vi "LineStyle_GetObjectStatus.vi"(0 "reference":refnum<class "LineStyle.lvclass">, 5 "error in (no error)":errorcluster) -> (14 "reference out":refnum<class "LineStyle.lvclass">, 16 "Type(String)":string, 19 "error out":errorcluster)   [LabVIEW 2020, in "LineStyle.lvclass"]
doc: "Gets an object"
uses:
  <resource>/Framework/Providers/Open_GDS/UML/LineStyle_class/LineStyle.lvclass
  <resource>/Framework/Providers/Open_GDS/UML/LineStyle_class/LineStyle.lvclass/LineStyle.ctl
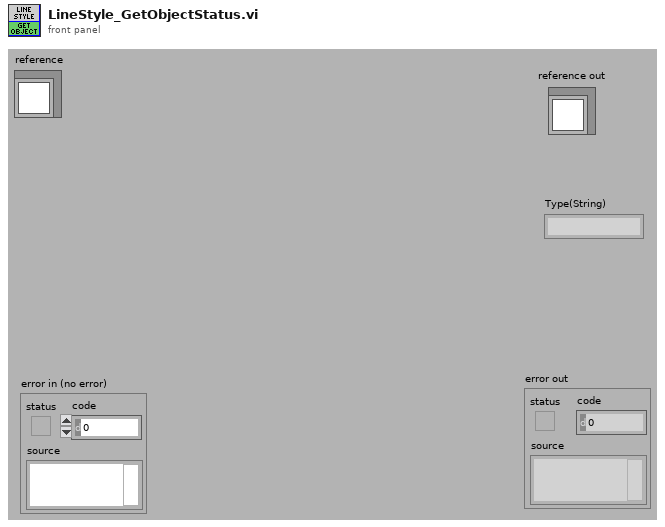
[diagram p1: front panel]
types:
  T1 = typedef "LineStyle.lvclass/LineStyleType.ctl" = enum16{"SOLID", "DOTTED"}
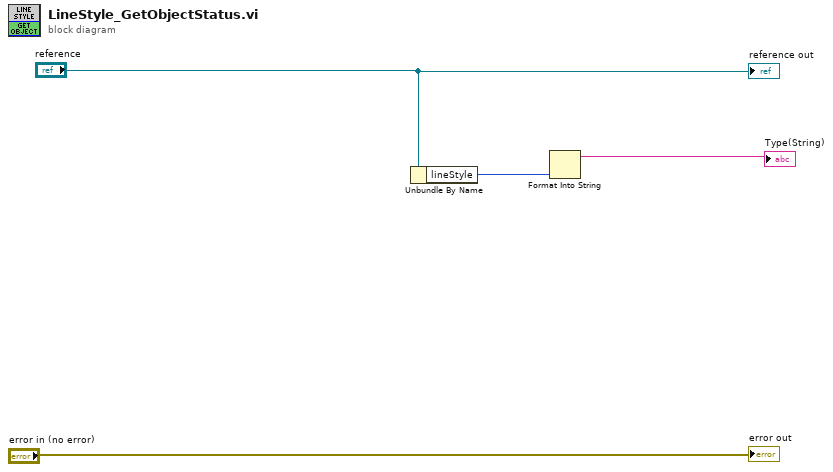
[diagram p0: block diagram]
diagram:
  n1 = Unbundle By Name("reference") -> ("lineStyle"=w3:T1)
  n2 = Format Into String(w3) -> (resulting string=→"Type(String)":string)  [unwired: 3 in, 1 out]
  "reference out" <- "reference"
  "error out" <- "error in (no error)"
